vi "Command cluster flatten VEPS LB.vi"(0 "command":T1) -> (1 "data string":string, 2 "type string":i16[](array[numeric])=[512, 16464, 7, 70, 80, 16, 4, 33, 4, 33, 4, 33, 4, 33, 4, 33, 4, 33, 4, 33, 4, 33, 4, 33, 4, 33, 4, 33, 4, 33, 4, 33, 4, 33, 4, 33, 4, 33, 70, 80, 16, 4, 33, 4, 33, 4, 33, 4, 33, 4, 33, 4, 33, 4, 33, 4, 33, 4, 33, 4, 33, 4, 33, 4, 33, 4, 33, 4, 33, 4, 33, 4, 33, 70, 80, 16, 4, 33, 4, 33, 4, 33, 4, 33, 4, 33, 4, 33, 4, 33, 4, 33, 4, 33, 4, 33, 4, 33, 4, 33, 4, 33, 4, 33, 4, 33, 4, 33, 70, 80, 16, 4, 33, 4, 33, 4, 33, 4, 33, 4, 33, 4, 33, 4, 33, 4, 33, 4, 33, 4, 33, 4, 33, 4, 33, 4, 33, 4, 33, 4, 33, 4, 33, 70, 80, 16, 4, 33, 4, 33, 4, 33, 4, 33, 4, 33, 4, 33, 4, 33, 4, 33, 4, 33, 4, 33, 4, 33, 4, 33, 4, 33, 4, 33, 4, 33, 4, 33, 70, 80, 16, 4, 33, 4, 33, 4, 33, 4, 33, 4, 33, 4, 33, 4, 33, 4, 33, 4, 33, 4, 33, 4, 33, 4, 33, 4, 33, 4, 33, 4, 33, 4, 33, 70, 80, 16, 4, 33, 4, 33, 4, 33, 4, 33, 4, 33, 4, 33, 4, 33, 4, 33, 4, 33, 4, 33, 4, 33, 4, 33, 4, 33, 4, 33, 4, 33, 4, 33, 3695, 30068, 28789, 29728, 25452, 30067, 29797, 29184])   [LabVIEW 2011]
panel:
  out "length":i32
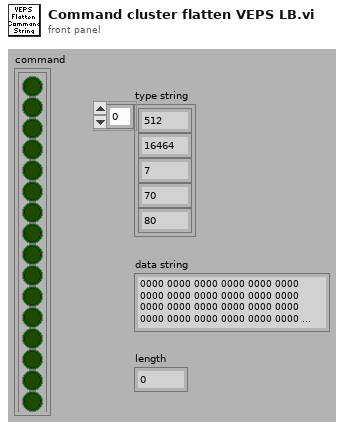
[diagram p1: front panel]
types:
  T1 = cluster{cluster{bool, bool, bool, bool, bool, bool, bool, bool, bool, bool, bool, bool, bool, bool, bool, bool}, cluster{bool, bool, bool, bool, bool, bool, bool, bool, bool, bool, bool, bool, bool, bool, bool, bool}, cluster{bool, bool, bool, bool, bool, bool, bool, bool, bool, bool, bool, bool, bool, bool, bool, bool}, cluster{bool, bool, bool, bool, bool, bool, bool, bool, bool, bool, bool, bool, bool, bool, bool, bool}}
  T2 = cluster{bool, bool, bool, bool, bool, bool, bool, bool, bool, bool, bool, bool, bool, bool, bool, bool}
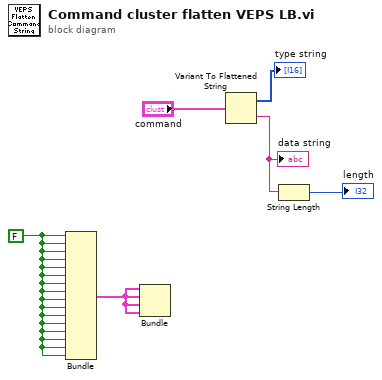
[diagram p0: block diagram]
diagram:
  w5 = FALSE
  n1 = Bundle(w5, w5, w5, w5, w5, w5, w5, w5, w5, w5, w5, w5, w5, w5, w5, w5) -> (w4:T2)  [unwired: 1 in]
  n2 = Bundle(w4, w4, w4, w4) -> ()  [unwired: 1 in, 1 out]
  n3 = Variant To Flattened String(Variant="command") -> (data string=w2:string, 1:→"type string":i16[])
  "data string" <- w2
  n4 = String Length(string=w2) -> (length=→"length":i32)
